vi "AG33XXX.set trigger.vi"(0 "i ref in":refnum<vi>, 2 "triggerParameters":i16[](array[numeric]), 3 "ms timeout (10000)":i32=10000, 5 "error in (no error)":errorcluster) -> (14 "i ref out":refnum<vi>, 17 "timed out":bool, 19 "error out":errorcluster)   [LabVIEW 2014, in "AG33XXX.lvlib"]
doc: "Sets the trigger parameters at my device."
uses:
  AG33XXX.lvlib
  CSCore/CSApplicationBaseClasses/AFGBase/AFGBase.serviceType.ctl
  CSCore/CSApplicationBaseClasses/AFGBase/AFGBase.directionType.ctl
  CSlibraries/UtilityLib/UtilityLib.valueStatus.ctl
  CSCore/CSApplicationBaseClasses/DeviceBase/DeviceBase.lvlib
  CSCore/CSApplicationBaseClasses/AFGBase/AFGBase.lvlib
  CSlibraries/UtilityLib/UtilityLib.lvlib
  CSinstr.lib/Agilent 33xxx Series/Agilent 33XXX Series.lvlib
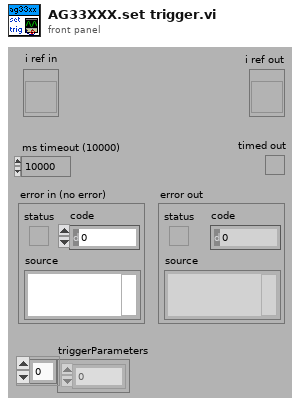
[diagram p1: front panel]
types:
  T1 = typedef "UtilityLib.lvlib/UtilityLib.valueStatus.ctl" = enum16{"no info available", "stand by/off", "on", "warning", "alarm/malfunction", "not implemented", "user action required", "important information", "system default", "control default", "indicator default", "button default"}
  T2 = typedef "AFGBase.lvlib/AFGBase.directionType.ctl" = enum16{"unknown", "update actual value", "update nominal value", "update both"}
  T3 = typedef "AFGBase.lvlib/AFGBase.serviceType.ctl" = enum16{"frequency", "amplitude", "phase", "DCOffset", "enableOutput", "trigger", "waveformType"}
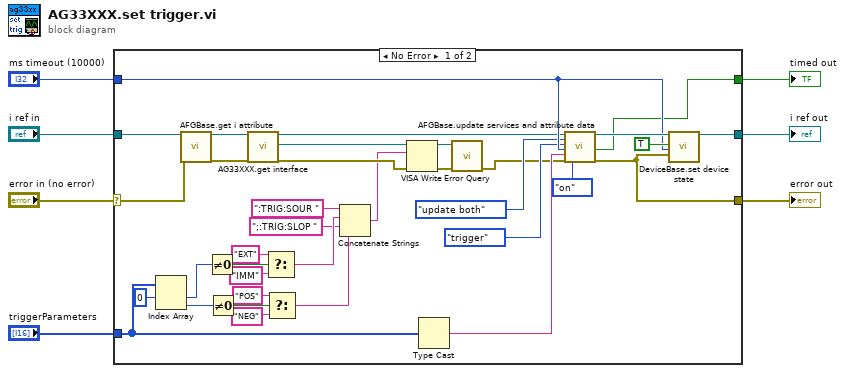
[diagram p0: block diagram]
diagram:
  n1 = case shown="No Error" "error in (no error)" {
    selector: "error in (no error)" -> [w32 w43]
    tunnel: [w42 w44] -> w7
    tunnel: "ms timeout (10000)" -> [w38 _]
    tunnel: "i ref in" -> [w33 w44]
    tunnel: [w39 w43] -> w3
    tunnel: "triggerParameters" -> [w24 _]
    tunnel: [w8 _] -> w1
    frame No Error {
      n2 = Index Array(array=w24, index #1=0 ("index")) -> (element #1=w21:i16, element #2=w15:i16)  [unwired: 1 in]
      n3 = call "AFGBase.get i attribute.vi"("i ref in"=w33, "error in (no error)"=w32) -> ("i ref out"=w30:refnum<vi>, "error out"=w31:errorcluster)  [unwired: 15 in, 1 out]
      n4 = Not Equal To 0?(x=w21) -> (x != 0?=w20:bool)
      n5 = Not Equal To 0?(x=w15) -> (x != 0?=w16:bool)
      n6 = call "AG33XXX.get interface.vi"("i ref in"=w30, "error in (no error)"=w31) -> ("i ref out"=w29:refnum<vi>, "interface"=w26:refnum<visa-resource-name>, "error out"=w25:errorcluster)  [unwired: 15 in]
      n7 = Select(t="EXT", s=w20, f="IMM") -> (s? t:f=w13:string)
      n8 = Select(t="POS", s=w16, f="NEG") -> (s? t:f=w11:string)
      n9 = Concatenate Strings(":TRIG:SOUR " ("string"), w13, ";:TRIG:SLOP " ("string"), w11) -> (w10:string)
      n10 = VISA Write(VISA resource name=w26, write buffer=w10, error in (no error)=w25) -> (VISA resource name out=w27:refnum<visa-resource-name>, error out=w28:errorcluster)  [unwired: 1 out]
      n11 = Type Cast(x=w24) -> (*(type *) &x=w36:string)  [unwired: 1 in]
      n12 = call "Error Query.vi"("error in (no error)"=w28, "VISA resource name"=w27) -> ("error out"=w22:errorcluster)  [unwired: 6 in, 3 out]
      n13 = call "AFGBase.update services and attribute data.vi"("i ref in"=w29, "direction"=AFGBase.directionType."update both", "service"=AFGBase.serviceType."trigger", "ms timeout (10000)"=w38, "value"=w36, "error in (no error)"=w22, "quality"=UtilityLib.valueStatus."on") -> ("i ref out"=w40:refnum<vi>, "timed out"=w8:bool, "error out"=w39:errorcluster)  [unwired: 10 in]
      n14 = call "DeviceBase.set device state.vi"("i ref in"=w40, "implicit"=TRUE, "ms timeout (10000)"=w38, "device error"=w39) -> ("i ref out"=w42:refnum<vi>)  [unwired: 13 in, 2 out]
    }
    frame Error {
    }
  }
  "error out" <- w3
  "i ref out" <- w7
  "timed out" <- w1
